vi "From JSON Text (string).vi"(7 "Data Type (default value)":string, 9 "error in (no error)":errorcluster, 10 "Offset":i32, 11 "JSON":string) -> (1 "error out":errorcluster, 2 "Offset past match":i32, 3 "String":string)   [LabVIEW 2019, in "JSONtext.lvlib"]
doc: "Convert the JSON Value at Offset into a LabVIEW type."
uses:
  JSONtext.lvlib
  support/Get String.vi
  Parsing/Advance past String.vi
  String Subset.vi
  support/Strip Quotes and Unescape.vi
  support/Unescape JSON string.vi
  Parsing/Parsing Error in converting to LabVIEW type.vi
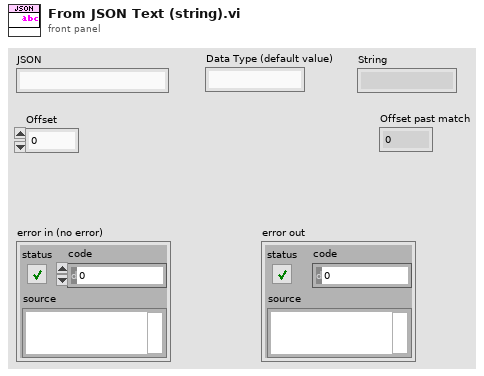
[diagram p1: front panel]
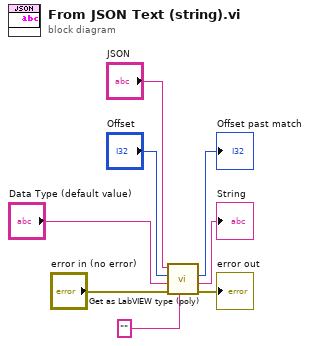
[diagram p0: block diagram]
diagram:
  n1 = call-poly "Get as LabVIEW type (poly).vi"("LV Type"="", "error in (no error)"="error in (no error)", "Data Type (default value)"="Data Type (default value)", "Offset"="Offset", "JSON"="JSON") -> ("error out"=→"error out":errorcluster, "String"=→"String":string, "Offset past match"=→"Offset past match":i32)  [unwired: 4 in]
